vi "Action Stop Heating.vi"(8 "error in (no error)":errorcluster, 11 "heater_parent in":refnum<class "heater_parent.lvclass">) -> (0 "error out":errorcluster, 3 "heater_parent out":refnum<class "heater_parent.lvclass">)   [LabVIEW 2020, in "polar_bear_plus_drivers.lvlib" / "heater_parent.lvclass"]
doc: "\"Stops\" the temperature controller by setting the setpoint to 25 Celsius. The previous setpoint is stored so you can \"resume\" heating when the \"start\" command is executed. This previous setpoint is not retained between sessions.\n\nThere is not a programmatic way to stop heading, as it is controlled by a switch on the side of the Polar Bear device. The best we can do is set the temperature to 25 Celsius so it is not dangerous."
uses:
  <instrlib>/RxnRover/Driver Polar Bear Plus/heater_parent/heater_parent.lvclass
  <instrlib>/RxnRover/Driver Polar Bear Plus/heater_parent/heater_parent.lvclass/heater_parent.ctl
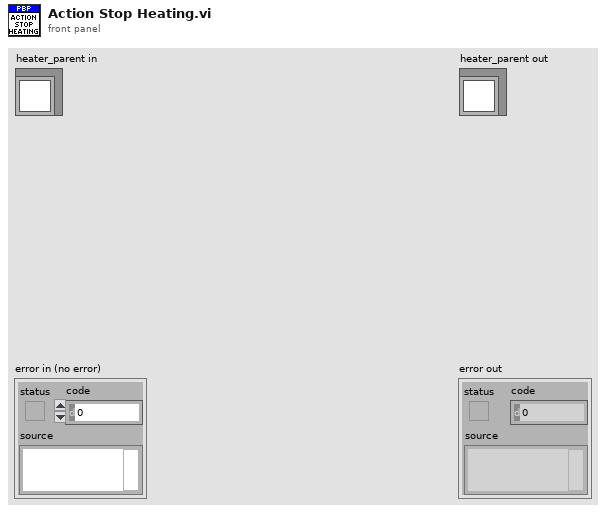
[diagram p1: front panel]
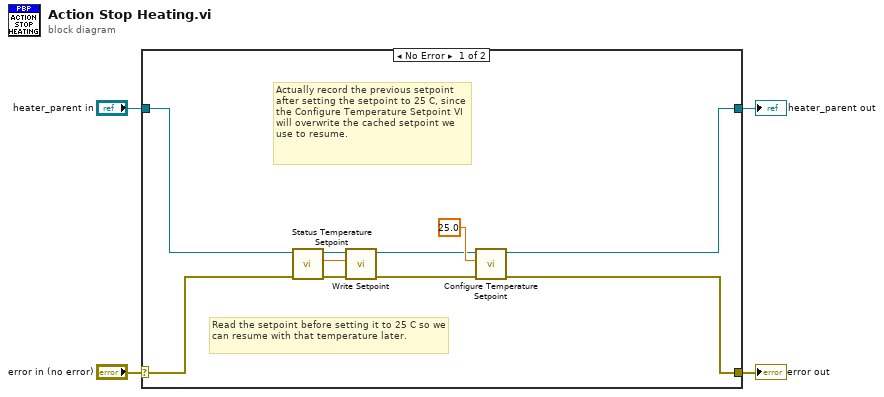
[diagram p0: block diagram]
diagram:
  n1 = case shown="No Error" "error in (no error)" {
    selector: "error in (no error)" -> [w11 w16]
    tunnel: [w14 w16] -> w3
    tunnel: [w13 w15] -> w1
    tunnel: "heater_parent in" -> [w12 w15]
    frame No Error {
      # "Read the setpoint before setting it to 25 C so we can resume with that temperature later."
      # "Actually record the previous setpoint after setting the setpoint to 25 C, since the Configure Temperature Setpoint VI will overwrite the cached setpoint we use to resume."
      n2 = call-dynamic "Status Temperature Setpoint.vi"("error in (no error)"=w11, "heater_parent in"=w12) -> ("error out"=w10:errorcluster, "Setpoint"=w5:dbl, "heater_parent out"=w7:refnum<class "heater_parent.lvclass">)  [unwired: 7 in]
      n3 = call-dynamic "Write Setpoint.vi"("error in (no error)"=w10, "Setpoint"=w5, "heater_parent in"=w7) -> ("error out"=w8:errorcluster, "heater_parent out"=w6:refnum<class "heater_parent.lvclass">)  [unwired: 7 in]
      n4 = call-dynamic "Configure Temperature Setpoint.vi"("error in (no error)"=w8, "New Setpoint"=25.0, "heater_parent in"=w6) -> ("error out"=w14:errorcluster, "heater_parent out"=w13:refnum<class "heater_parent.lvclass">)  [unwired: 7 in]
    }
    frame Error {
    }
  }
  "error out" <- w3
  "heater_parent out" <- w1
